vi "Scan for Pumps.vi"(8 "error in (no error)":errorcluster, 11 "ASIA Pump # In":i32) -> (0 "error out":errorcluster, 2 "pumpCnt":u32, 3 "ASIA Pump # Out":i32)   [LabVIEW 2018, in "ASIA Pump.lvlib"]
uses:
  ASIA Pump.lvlib
panel:
  out "path out":path
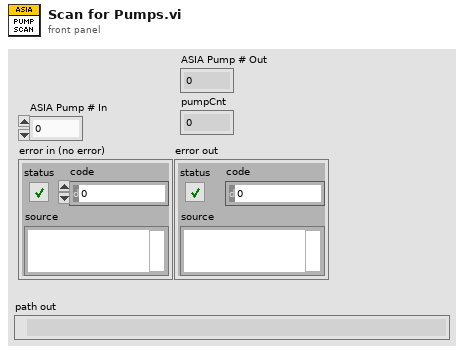
[diagram p1: front panel]
types:
  T1 = cluster{"Busy":bool, "PumpCnt":dbl, "RemoteEntered":bool, "OverpressureSet":bool}[]
  T2 = cluster{"Busy":bool, "PumpCnt":dbl, "RemoteEntered":bool, "OverpressureSet":bool}
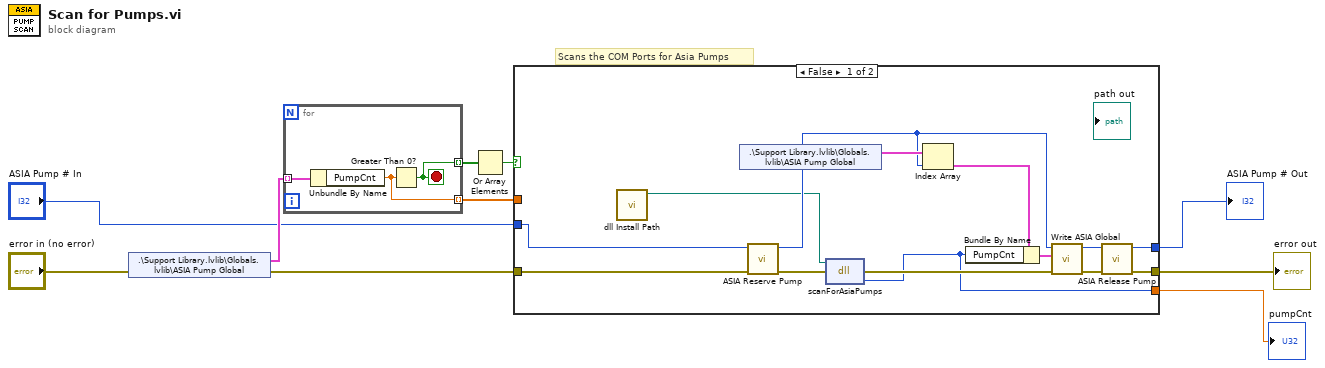
[diagram p0: block diagram]
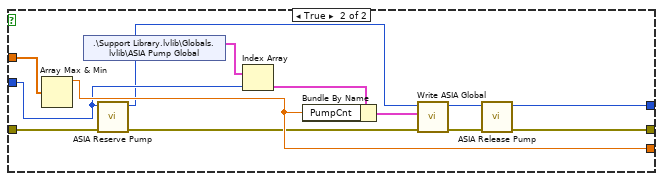
[diagram p2: hidden frame]
diagram:
  # "Scans the COM Ports for Asia Pumps"
  n1 = shared-variable ".\\Support Library.lvlib\\Globals.lvlib\\ASIA Pump Global"(error in="error in (no error)") -> (w10:T1, error out=w1:errorcluster)
  n2 = for {
    tunnel: w10 -> [w13] mode=indexing
    tunnel: [w12] -> w9 mode=indexing
    tunnel: [w11] -> w4 mode=indexing
    stop <- w12 stop-if-true
    n3 = Unbundle By Name(w13) -> ("PumpCnt"=w11:dbl)
    n4 = Greater Than 0?(x=w11) -> (x > 0?=w12:bool)
  }
  n5 = Or Array Elements(Boolean array=w9) -> (logical OR=w8:bool)
  n6 = case shown="False" w8 {
    tunnel: w1 -> [w25 w31]
    tunnel: "ASIA Pump # In" -> [w24 w30]
    tunnel: [w16 w32] -> w3
    tunnel: [w15 w33] -> w6
    tunnel: [w22 w36] -> w5
    tunnel: w4 -> [_ w40]
    frame False {
      n7 = call "dll Install Path.vi"() -> ("system directory"=w14:path)  [unwired: 11 in]
      n8 = shared-variable ".\\Support Library.lvlib\\Globals.lvlib\\ASIA Pump Global"() -> (w21:T1)  [unwired: 1 in, 1 out]
      n9 = call "ASIA Reserve Pump.vi"("error in (no error)"=w25, "ASIA Pump # In"=w24) -> ("error out"=w27:errorcluster, "ASIA Pump # Out"=w20:i32)  [unwired: 8 in]
      n10 = dll-call lib="C:/Program Files (x86)/Pfizer/FAST/data/AsiaPumpInterface.dll" fn="scanForAsiaPumps"(path in=w14, error in=w27) -> (error out=w26:errorcluster, "pumpCnt"=w22:u32)  [unwired: 1 in, 1 out]
      n11 = Index Array(array=w21, index=w20) -> (element=w19:T2)
      n12 = Bundle By Name(cluster=w19, "PumpCnt"=w22) -> (w23:T2)
      n13 = call "Write ASIA Global.vi"("error in (no error)"=w26, "ASIA Global"=w23, "Pump Number In"=w20) -> ("error out"=w17:errorcluster, "Pump Number Out"=w18:i32)  [unwired: 7 in]
      n14 = call "ASIA Release Pump.vi"("error in (no error)"=w17, "pumpNum"=w18) -> ("error out"=w16:errorcluster, "ASIA Pump # Out"=w15:i32)  [unwired: 8 in]
    }
    frame True {
      n15 = Array Max & Min(array=w40) -> (max value=w36:dbl)  [unwired: 3 out]
      n16 = shared-variable ".\\Support Library.lvlib\\Globals.lvlib\\ASIA Pump Global"() -> (w38:T1)  [unwired: 1 in, 1 out]
      n17 = call "ASIA Reserve Pump.vi"("error in (no error)"=w31, "ASIA Pump # In"=w30) -> ("error out"=w28:errorcluster, "ASIA Pump # Out"=w29:i32)  [unwired: 8 in]
      n18 = Index Array(array=w38, index=w30) -> (element=w37:T2)
      n19 = Bundle By Name(cluster=w37, "PumpCnt"=w36) -> (w39:T2)
      n20 = call "Write ASIA Global.vi"("error in (no error)"=w28, "ASIA Global"=w39, "Pump Number In"=w29) -> ("error out"=w35:errorcluster, "Pump Number Out"=w34:i32)  [unwired: 7 in]
      n21 = call "ASIA Release Pump.vi"("error in (no error)"=w35, "pumpNum"=w34) -> ("error out"=w32:errorcluster, "ASIA Pump # Out"=w33:i32)  [unwired: 8 in]
    }
  }
  "ASIA Pump # Out" <- w6
  "pumpCnt" <- w5
  "error out" <- w3
